vi "Measurement-CT.vi"(8 "Numeric":dbl, 9 "Cluster 2":T1={"客户仪器地址"="USB0::0x0471::0x2826::QF71600867::INSTR", "BSFR"=refnum, "测试频率"=100000.0, "error in (no error)"={"status"=FALSE, "code"=0, "source"=""}}, 10 "Ctl Refnum 2":refnum<vi>, 11 "Ctl Refnum":refnum<vi>) -> (1 "Cluster":T2)   [LabVIEW 2017]
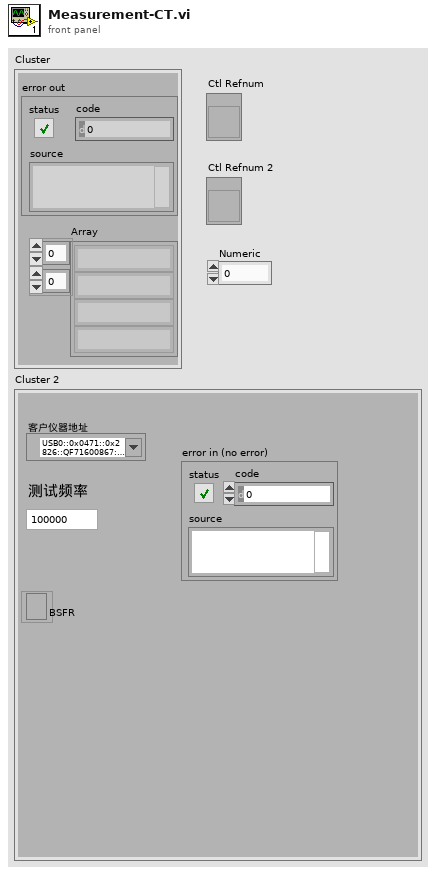
[diagram p1: front panel]
types:
  T1 = cluster{"客户仪器地址":refnum<visa-resource-name>, "BSFR":refnum<file>, "测试频率":dbl, "error in (no error)":errorcluster}
  T2 = cluster{"Array":string[][], "error out":errorcluster}
  T3 = cluster{"Array 2":string[][], "error out":errorcluster}
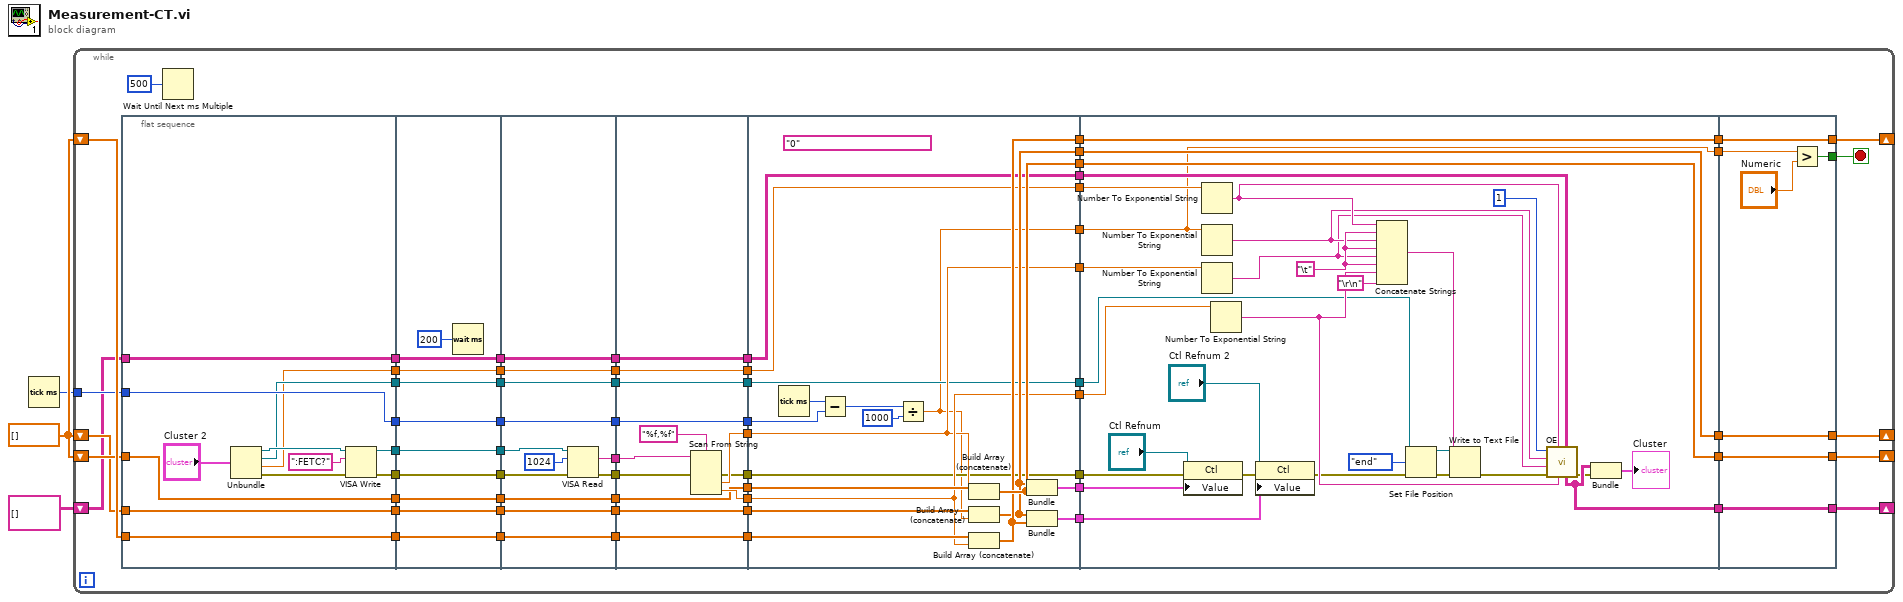
[diagram p0: block diagram]
diagram:
  w3 = dbl[] []
  n1 = Tick Count (ms)() -> (millisecond timer value=w1:u32)
  n2 = while {
    tunnel: w1 -> [w17]
    shift-right: [w15] -> _
    shift-left: w3 -> [w20]
    shift-right: [w10] -> _
    shift-left: w3 -> [w18]
    shift-right: [w14] -> _
    shift-left: w3 -> [w19]
    shift-right: [w13] -> _
    shift-left: string[][] [] -> [w16]
    stop <- w4 stop-if-true
    n3 = flat-sequence {
      tunnel: w20 -> [w78]
      tunnel: w19 -> [w79]
      tunnel: w18 -> [w80]
      tunnel: w17 -> [w81]
      tunnel: [w81] -> w68
      tunnel: [w80] -> w67
      tunnel: [w79] -> w66
      tunnel: [w78] -> w65
      tunnel: [w76] -> w64
      tunnel: [w75] -> w63
      tunnel: [w74] -> w62
      tunnel: w16 -> [w74]
      tunnel: [w72] -> w61
      tunnel: [w71] -> w60
      tunnel: [w91] -> w59
      tunnel: [w90] -> w58
      tunnel: [w89] -> w57
      tunnel: [w88] -> w56
      tunnel: w68 -> [w91]
      tunnel: w67 -> [w90]
      tunnel: w66 -> [w89]
      tunnel: w65 -> [w88]
      tunnel: [w86] -> w55
      tunnel: w64 -> [w86]
      tunnel: [w85] -> w54
      tunnel: w63 -> [w85]
      tunnel: [w84] -> w53
      tunnel: w62 -> [w84]
      tunnel: [w83] -> w52
      tunnel: w61 -> [w83]
      tunnel: [w82] -> w51
      tunnel: w60 -> [w82]
      tunnel: [w103] -> w50
      tunnel: [w102] -> w49
      tunnel: [w101] -> w48
      tunnel: [w100] -> w47
      tunnel: [w97] -> w46
      tunnel: [w98] -> w45
      tunnel: w59 -> [w103]
      tunnel: w58 -> [w102]
      tunnel: w57 -> [w101]
      tunnel: w56 -> [w100]
      tunnel: w55 -> [w96]
      tunnel: w54 -> [w95]
      tunnel: [w94] -> w44
      tunnel: w53 -> [w94]
      tunnel: [w93] -> w43
      tunnel: w52 -> [w93]
      tunnel: w51 -> [w92]
      tunnel: [w92] -> w42
      tunnel: [w113] -> w41
      tunnel: [w112] -> w40
      tunnel: [w111] -> w39
      tunnel: [w110] -> w38
      tunnel: [w115] -> w37
      tunnel: [w114] -> w36
      tunnel: [w109] -> w35
      tunnel: w50 -> [w113]
      tunnel: w49 -> [w112]
      tunnel: w48 -> [w111]
      tunnel: w47 -> [w110]
      tunnel: w46 -> [w108]
      tunnel: w45 -> [w107]
      tunnel: [w106] -> w34
      tunnel: w44 -> [w106]
      tunnel: [w105] -> w33
      tunnel: w43 -> [w105]
      tunnel: [w104] -> w32
      tunnel: w42 -> [w104]
      tunnel: w41 -> [w134]
      tunnel: w40 -> [w132]
      tunnel: w39 -> [w131]
      tunnel: w38 -> [w130]
      tunnel: [w129] -> w31
      tunnel: [w128] -> w30
      tunnel: [w127] -> w29
      tunnel: w37 -> [w124]
      tunnel: [w124] -> w28
      tunnel: w36 -> [w125]
      tunnel: [w125] -> w27
      tunnel: [w117] -> w26
      tunnel: w35 -> [w123]
      tunnel: [w123] -> w25
      tunnel: w34 -> [w122]
      tunnel: [w122] -> w24
      tunnel: w33 -> [w118]
      tunnel: [w121] -> w23
      tunnel: w32 -> [w121]
      tunnel: [w120] -> w22
      tunnel: [w119] -> w21
      tunnel: [w118] -> w11
      tunnel: w31 -> [w161]
      tunnel: w30 -> [w160]
      tunnel: w29 -> [w159]
      tunnel: w28 -> [w138]
      tunnel: w27 -> [w158]
      tunnel: w26 -> [w136]
      tunnel: w25 -> [w149]
      tunnel: w24 -> [w156]
      tunnel: w23 -> [w139]
      tunnel: w22 -> [w148]
      tunnel: w21 -> [w147]
      tunnel: w11 -> [w141]
      tunnel: [w161] -> w9
      tunnel: [w160] -> w8
      tunnel: [w159] -> w7
      tunnel: [w151] -> w6
      tunnel: [w136] -> w5
      tunnel: [w170] -> w13
      tunnel: [w171] -> w10
      tunnel: [w172] -> w15
      tunnel: [w173] -> w14
      tunnel: w9 -> [w173]
      tunnel: w8 -> [w172]
      tunnel: w7 -> [w171]
      tunnel: w6 -> [w170]
      tunnel: w5 -> [w169]
      tunnel: [w167] -> w4
      frame #0 {
        n4 = Unbundle("Cluster 2") -> ("客户仪器地址"=w73:refnum<visa-resource-name>, "BSFR"=w72:refnum<file>, "测试频率"=w71:dbl, "error in (no error)"=w69:errorcluster)
        n5 = VISA Write(VISA resource name=w73, write buffer=":FETC?", error in (no error)=w69) -> (VISA resource name out=w76:refnum<visa-resource-name>, error out=w75:errorcluster)  [unwired: 1 out]
      }
      frame #1 {
        n6 = Wait (ms)(milliseconds to wait=u32 200 ("等待时间（毫秒）")) -> ()  [unwired: 1 out]
      }
      frame #2 {
        n7 = VISA Read(VISA resource name=w96, byte count=u32 1024 ("字节总数"), error in (no error)=w95) -> (read buffer=w97:string, error out=w98:errorcluster)  [unwired: 2 out]
      }
      frame #3 {
        n8 = Scan From String(format string="%f,%f" ("格式字符串"), input string=w108, error in=w107) -> (error out=w109:errorcluster, output 1=w115:dbl, output 2=w114:dbl)  [unwired: 3 in, 2 out]
      }
      frame #4 {
        (unwired) "0" ("Input Z format")
        n9 = Tick Count (ms)() -> (millisecond timer value=w135:u32)
        n10 = Subtract(x=w135, y=w134) -> (x-y=w133:u32)
        n11 = Divide(x=w133, y=u32 1000) -> (x/y=w117:dbl)
        n12 = Build Array (concatenate)(w131, w124) -> (w129:dbl[])
        n13 = Build Array (concatenate)(w132, w117) -> (w127:dbl[])
        n14 = Build Array (concatenate)(w130, w125) -> (w128:dbl[])
        n15 = Bundle(w127, w129) -> (w119:cluster{dbl[], dbl[]})  [unwired: 1 in]
        n16 = Bundle(w127, w128) -> (w120:cluster{dbl[], dbl[]})  [unwired: 1 in]
      }
      frame #5 {
        w162 = "\t"
        n17 = property class="Ctl"(reference="Ctl Refnum", error in=w149, "Value"=w147) -> (error out=w150:errorcluster)  [unwired: 1 out]
        n18 = Number To Exponential String(number=w139) -> (E-format string=w155:string)  [unwired: 3 out]
        n19 = Number To Exponential String(number=w136) -> (E-format string=w154:string)  [unwired: 3 out]
        n20 = Number To Exponential String(number=w138) -> (E-format string=w153:string)  [unwired: 3 out]
        n21 = Number To Exponential String(number=w158) -> (E-format string=w152:string)  [unwired: 3 out]
        n22 = property class="Ctl"(reference="Ctl Refnum 2", error in=w150, "Value"=w148) -> (error out=w140:errorcluster)  [unwired: 1 out]
        n23 = Concatenate Strings(w155, w162, w154, w162, w153, w162, w152, "\r\n") -> (w164:string)
        n24 = Set File Position(refnum=w141, from (0:start)=enum16{"start", "end", "current"}."end" ("自（0:起始）"), error in=w140) -> (refnum out=w166:refnum<file>, error out=w163:errorcluster)  [unwired: 1 out]
        n25 = Write to Text File(file (use dialog)=w166, text=w164, error in=w163) -> (error out=w143:errorcluster)  [unwired: 3 out]
        n26 = call "OE.vi"("Array"=w156, "String 4"=w152, "String"=w155, "error in (no error)"=w143, "String 3"=w153, "String 2"=w154, "Numeric"=1) -> ("error out"=w142:errorcluster, "Array 2"=w151:string[][])  [unwired: 2 in, 1 out]
        n27 = Bundle("Array 2"=w151, "error out"=w142) -> (→"Cluster":T3)  [unwired: 1 in]
      }
      frame #6 {
        n28 = Greater?(x=w169, y="Numeric") -> (0:w167:bool)
      }
    }
    n29 = Wait Until Next ms Multiple(millisecond multiple=u32 500 ("毫秒倍数")) -> ()  [unwired: 1 out]
  }
